vi "simplePID_antiwindup.vi"(0 "setpoint":i16, 1 "reset? (F)":bool, 2 "Input Selector":u8, 3 "channel (0)":u8, 5 "process variable":i16, 7 "manual control":T3, 12 "Gains":T1, 13 "output range":T5={"output high (Inf)"=inf, "output low (-Inf)"=-inf}, 14 "setpoint weighting":T4={"proportional weighting (1)"=1.0, "derivative weighting (0)"=0.0} {"derivative weighting (0)" min=0 max=1; "proportional weighting (1)" min=0 max=1}) -> (4 "output":sgl, 6 "error":sgl, 8 "actions":T2)   [LabVIEW 2020]
uses:
  <vilib>/rvi/Analysis/control/PID/Typedef/niFpgaPID_PIDErrors.ctl
  Typedef/niFpgaPID_OutputRange.ctl
  Typedef/niFpgaPID_SetpointWeightings.ctl
  Typedef/niFpgaPID_ManualControl.ctl
  Typedef/niFpgaPID_PIDActions.ctl
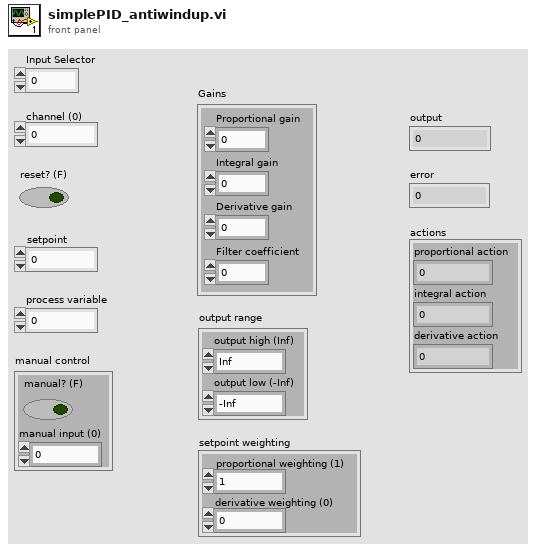
[diagram p1: front panel]
types:
  T1 = cluster{"Proportional gain":sgl, "Integral gain":sgl, "Derivative gain":sgl, "Filter coefficient":sgl}
  T2 = typedef "niFpgaPID_PIDActions.ctl" = cluster{"proportional action":sgl, "integral action":sgl, "derivative action":sgl}
  T3 = typedef "niFpgaPID_ManualControl.ctl" = cluster{"manual? (F)":bool, "manual input (0)":sgl}
  T4 = typedef "niFpgaPID_SetpointWeightings.ctl" = cluster{"proportional weighting (1)":sgl, "derivative weighting (0)":sgl}
  T5 = typedef "niFpgaPID_OutputRange.ctl" = cluster{"output high (Inf)":sgl, "output low (-Inf)":sgl}
  T6 = typedef "niFpgaPID_PIDErrors.ctl" = cluster{"error":sgl, "error with beta":sgl, "error with gamma":sgl}
  T7 = typedef "niFpgaPID_PIDState.ctl" = cluster{"uI(k-1)":sgl, "e(k-1)":sgl, "e(k-1) with gamma":sgl, "output (k-1)":sgl, "uD(k-1)":sgl}
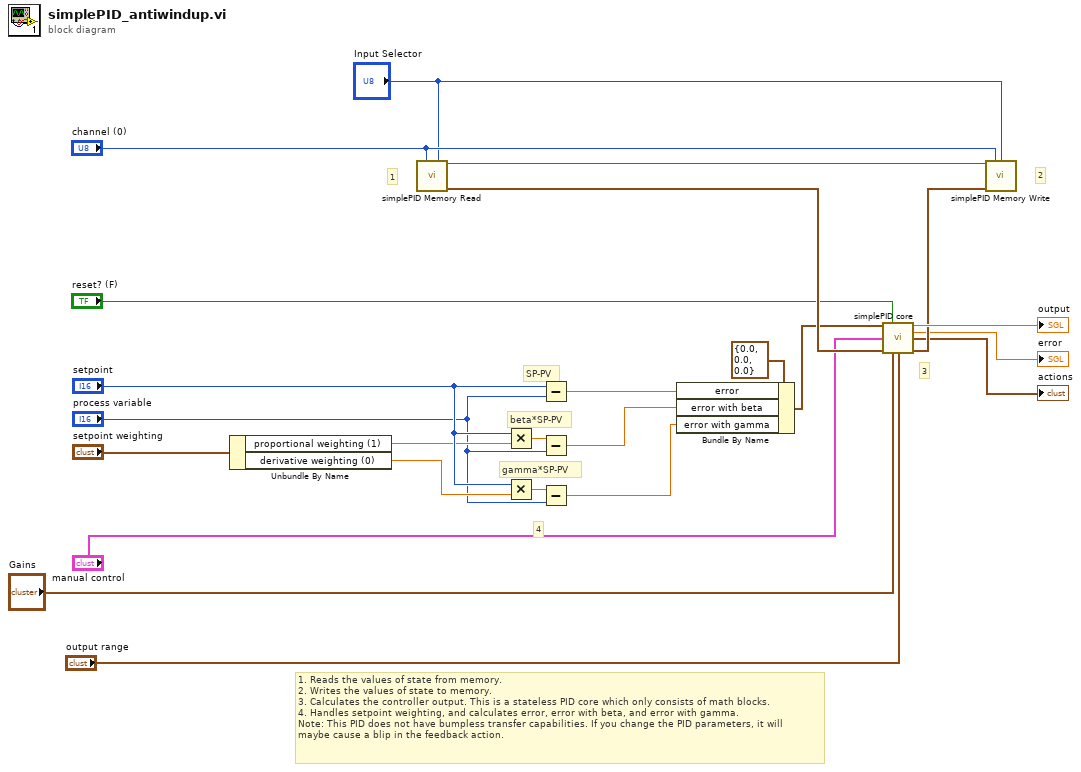
[diagram p0: block diagram]
diagram:
  # "SP-PV"
  # "beta*SP-PV"
  # "gamma*SP-PV"
  # "1. Reads the values of state from memory.\n2. Writes the values of state to memory.\n3. Calculates the controller output. This is a stateless PID core which only consists of math blocks.\n4. Handles setpoint weighting, and calculates error, error with beta, and error with gamma.\nNote: This PID does not have bumpless transfer capabilities. If you change the PID parameters, it will\nmaybe cause a blip in the feedback action."
  # "4"
  # "3"
  # "2"
  # "1"
  n1 = Unbundle By Name("setpoint weighting") -> ("proportional weighting (1)"=w16:sgl, "derivative weighting (0)"=w22:sgl)
  n2 = call "simplePID Memory Read.vi"("channel (0)"="channel (0)", "Input Selector"="Input Selector") -> ("memory out"=w2:refnum<k21>, "state out"=w20:T7)  [unwired: 12 in]
  n3 = Multiply(x="setpoint", y=w16) -> (x*y=w4:sgl)
  n4 = Multiply(x="setpoint", y=w22) -> (x*y=w5:sgl)
  n5 = Subtract(x="setpoint", y="process variable") -> (x-y=w8:sgl)
  n6 = Subtract(x=w4, y="process variable") -> (x-y=w13:sgl)
  n7 = Subtract(x=w5, y="process variable") -> (x-y=w12:sgl)
  n8 = Bundle By Name(cluster=T6 {"error"=0.0, "error with beta"=0.0, "error with gamma"=0.0} ("errors"), "error"=w8, "error with beta"=w13, "error with gamma"=w12) -> (w11:T6)
  n9 = call "simplePID core.vi"("errors"=w11, "reset? (F)"="reset? (F)", "manual control"="manual control", "state in"=w20, "gains"="Gains", "output range"="output range") -> ("output"=→"output":sgl, "error"=→"error":sgl, "actions"=→"actions":T2, "state out"=w21:T7)  [unwired: 6 in]
  n10 = call "simplePID Memory Write.vi"("memory in"=w2, "channel (0)"="channel (0)", "Input Selector"="Input Selector", "state in"=w21) -> ()  [unwired: 12 in]
